vi "Configure Eres.vi"(6 "Enable Eres Mode (T: Enable)":bool=TRUE, 7 "Source (0: Channel 1)":u16(ring) items=["Channel 1", "Channel 2", "Channel 3", "Channel 4", "Memory 1", "Memory 2", "Memory 3", "Memory 4", "Function 1", "Function 2", "Function 3", "Function 4", "Function 5", "Function 6", "Function 7", "Function 8"], 8 "error in (no error)":errorcluster, 9 "ERES Bits (0: 0.5)":u16(ring) items=["0.5", "1", "1.5", "2", "2.5", "3"], 10 "Target (0: Function 1)":u16(ring) items=["Function 1", "Function 2", "Function 3", "Function 4", "Function 5", "Function 6", "Function 7", "Function 8"], 11 "VISA resource name":refnum<visa-resource-name>) -> (0 "error out":errorcluster, 3 "VISA resource name out":refnum<visa-resource-name>)   [LabVIEW 2013, in "LeCroy Wave Series.lvlib"]
doc: "ERES (Enhanced Resolution) filtering increases vertical resolution, allowing you to distinguish closely spaced voltage levels. The functioning of the instrument's ERES is similar to smoothing the signal with a simple, moving-average filter. However, it is more efficient concerning bandwidth and pass-band filtering. Use ERES on single-shot waveforms, or where the data record is slowly repetitive (when you cannot use averaging). Use it to reduce noise when your signal is noticeably noisy, but you do not need to perform noise measurements. Also use it when you perform high precision voltage measurements: zooming with high vertical gain, for example."
uses:
  LeCroy Wave Series.lvlib
panel:
  # "Enable\n\nDisable"
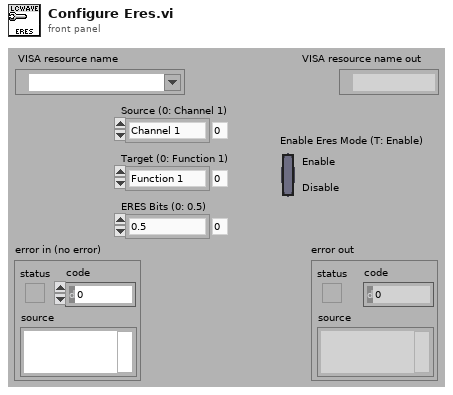
[diagram p1: front panel]
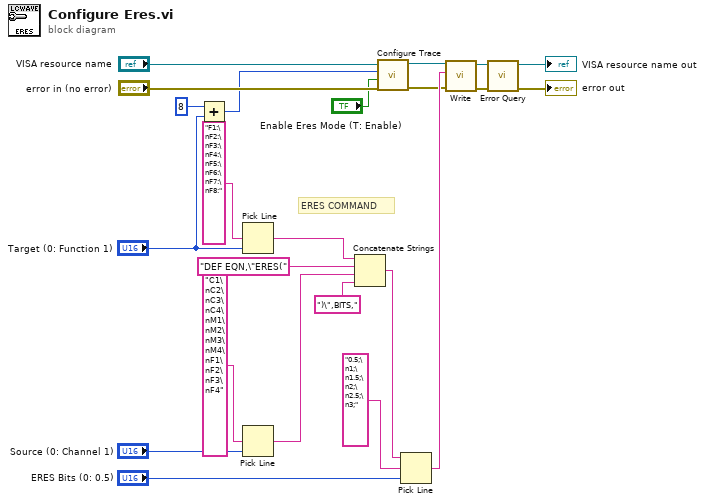
[diagram p0: block diagram]
diagram:
  # "ERES COMMAND"
  n1 = Add(x=u16 8, y="Target (0: Function 1)") -> (x+y=w4:u16)
  n2 = Pick Line(multi-line string="F1:\nF2:\nF3:\nF4:\nF5:\nF6:\nF7:\nF8:", line index="Target (0: Function 1)") -> (output string=w16:string)  [unwired: 1 in]
  n3 = Pick Line(multi-line string="C1\nC2\nC3\nC4\nM1\nM2\nM3\nM4\nF1\nF2\nF3\nF4", line index="Source (0: Channel 1)") -> (output string=w14:string)  [unwired: 1 in]
  n4 = Concatenate Strings(w16, "DEF EQN,\"ERES(", w14, ")\",BITS,") -> (w10:string)
  n5 = call "Configure Trace.vi"("error in (no error)"="error in (no error)", "Enable Trace Mode (T: Enable)"="Enable Eres Mode (T: Enable)", "Trace (0: Channel 1)"=w4, "VISA resource name"="VISA resource name") -> ("error out"=w5:errorcluster, "VISA resource name out"=w6:refnum<visa-resource-name>)  [unwired: 6 in]
  n6 = Pick Line(string ("")=w10, multi-line string="0.5;\n1;\n1.5;\n2;\n2.5;\n3;", line index="ERES Bits (0: 0.5)") -> (output string=w9:string)
  n7 = call "Write.vi"("error in (no error)"=w5, "Write Buffer"=w9, "VISA resource name"=w6) -> ("error out"=w20:errorcluster, "VISA resource name out"=w21:refnum<visa-resource-name>)  [unwired: 6 in, 1 out]
  n8 = call "Error Query.vi"("error in (no error)"=w20, "VISA resource name"=w21) -> ("error out"=→"error out":errorcluster, "VISA resource name out"=→"VISA resource name out":refnum<visa-resource-name>)  [unwired: 6 in, 2 out]
